vi "UI_AutoRefresh_Do.vi"(8 "error in (no error)":errorcluster, 9 "Parameters":T1={"Write TipStrips with details (T)"=TRUE, "Write Captions with UserLabels (T)"=TRUE, "Mode (ind only)"=enum."Indicators only", "Enable nested stream (T)"=TRUE}, 10 "Databox_sealed":refnum<class "Databox_sealed.lvclass">, 11 "LiveDatActor in":refnum<class "LiveDatActor.lvclass">) -> (0 "error out":errorcluster, 3 "LiveDatActor out":refnum<class "LiveDatActor.lvclass">)   [LabVIEW 2020, in "LiveDatActor.lvlib" / "LiveDatActor.lvclass"]
doc: "Enable nested stream : Permet le routage de la databox vers les nested UIA de l'acteur. On peut couper ce ruissellement si les nested n'ont pas besoin de databox pour optimiser le programme."
uses:
  LiveDatActor.lvclass
  support/UI_Actor.lvlibp/UI_Actor/ctl_AR_Parameters.ctl
  support/UI_Actor.lvlibp/UI_Actor/ctl_AR_Mode.ctl
  support/Databox.lvlibp/Databox_sealed/Databox_sealed.lvclass
  LiveDatActor.lvclass/LiveDatActor.ctl
  support/Databox.lvlibp/TypesTools/Data/Read Time.vi
  support/UI_Actor.lvlibp/UI_Actor/UI_Actor.lvclass
  support/Databox.lvlibp/TypesTools/Data/Data.lvclass
  D:/Projets/STEP AT/Bahamut/support/UI_Actor.lvlibp/UI_Actor/UI_Actor.lvclass
  D:/Projets/STEP AT/Bahamut/support/Actor Framework.lvlibp/1abvi3w/vi.lib/ActorFramework/Actor/Actor.lvclass
  D:/Projets/STEP AT/Bahamut/D&Cs/LiveDatActor/LiveDatActor/LiveDatActor.lvclass
  support/Databox.lvlibp/Databox/Databox.lvclass
  D:/Projets/STEP AT/Bahamut/support/Databox.lvlibp/Databox/Databox.lvclass
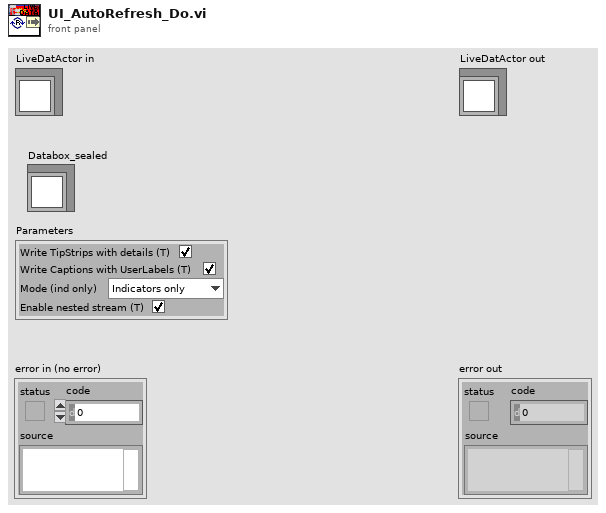
[diagram p1: front panel]
types:
  T1 = typedef "UI_Actor.lvlibp/UI_Actor.lvclass/ctl_AR_Parameters.ctl" = cluster{"Write TipStrips with details (T)":bool, "Write Captions with UserLabels (T)":bool, "Mode (ind only)":T2, "Enable nested stream (T)":bool}
  T2 = typedef "UI_Actor.lvlibp/UI_Actor.lvclass/ctl_AR_Mode.ctl" = enum16{"Controls only", "Indicators only", "All"}
  T3 = cluster{"Name":string, "Data":refnum<class "Data.lvclass">[]}[]
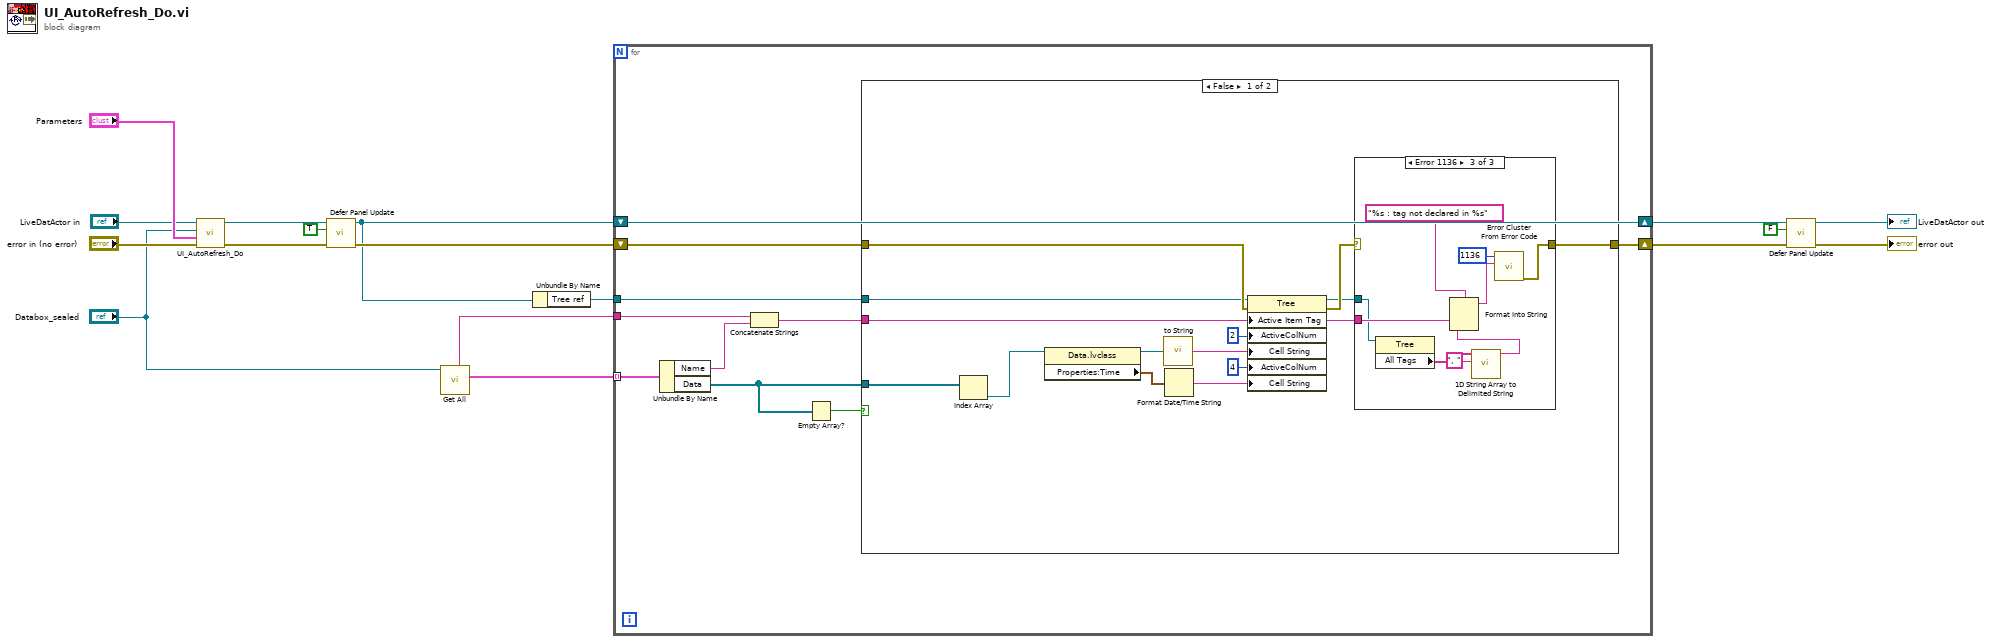
[diagram p0: block diagram]
diagram:
  n1 = call-parent "UI_AutoRefresh_Do.vi"("error in (no error)"="error in (no error)", "Parameters"="Parameters", "Databox_sealed"="Databox_sealed", "UI_Actor in"="LiveDatActor in") -> ("error out"=w11:errorcluster, "UI_Actor out"=w12:refnum<class "LiveDatActor.lvclass">)  [unwired: 6 in]
  n2 = call "Defer Panel Update.vi"("error in (no error)"=w11, "Defer Panel Updates"=TRUE, "UI_Actor in"=w12) -> ("error out"=w10:errorcluster, "UI_Actor out"=w9:refnum<class "LiveDatActor.lvclass">)  [unwired: 7 in]
  n3 = call "Get All.vi"("Databox in"="Databox_sealed") -> ("Names and data"=w2:T3, "Builder name"=w1:string)  [unwired: 5 in, 4 out]
  n4 = Unbundle By Name(w9) -> ("Tree ref"=w4:refnum<vi>)
  n5 = for {
    tunnel: w4 -> [w25]
    shift-right: [w27] -> w6
    shift-left: w9 -> [w27]
    shift-right: [w24] -> w8
    shift-left: w10 -> [w26]
    tunnel: w2 -> [w23] mode=indexing
    tunnel: w1 -> [w21]
    n6 = Unbundle By Name(w23) -> ("Name"=w20:string, "Data"=w19:refnum<class "Data.lvclass">[])
    n7 = Concatenate Strings(w21, w20) -> (w22:string)
    n8 = Empty Array?(array=w19) -> (empty?=w18:bool)
    n9 = case shown="False" w18 {
      tunnel: w26 -> [w41 w53]
      tunnel: w25 -> [w40 _]
      tunnel: [w39 w53] -> w24
      tunnel: w22 -> [w31 _]
      tunnel: w19 -> [w28 _]
      frame False {
        n10 = Index Array(array=w28) -> (element=w29:refnum<class "Data.lvclass">)  [unwired: 1 in]
        n11 = property class="Data.lvclass"(reference=w29) -> (reference out=w38:refnum<class "Data.lvclass">, "Properties:Time"=w34:timestamp)  [unwired: 1 in, 1 out]
        n12 = call "to String.vi"("Data"=w38) -> ("String"=w35:string)
        n13 = Format Date/Time String(seconds (now)=w34) -> (date/time string=w33:string)  [unwired: 2 in]
        n14 = property class="Tree"(reference=w40, error in=w41, "Active Item Tag"=w31, "ActiveColNum"=2 ("Active Cell:Active Column Number"), "Cell String"=w35, "ActiveColNum"=4 ("Active Cell:Active Column Number"), "Cell String"=w33) -> (reference out=w30:refnum<vi>, error out=w32:errorcluster)
        n15 = case shown="Error 1136" w32 {
          selector: w32 -> [w42 w43 _]
          tunnel: [w42 w43 w52] -> w39
          tunnel: w31 -> [_ _ w50]
          tunnel: w30 -> [_ _ w47]
          frame No Error {
          }
          frame Default {
          }
          frame Error {
            n16 = property class="Tree"(reference=w47) -> ("All Tags"=w46:string[])  [unwired: 1 in, 2 out]
            n17 = call <vilib>:"1D String Array to Delimited String.vi"("delimiter"=", ", "string array"=w46) -> ("delimited string"=w45:string)  [unwired: 9 in]
            n18 = Format Into String(format string="%s : tag not declared in %s", w50, w45) -> (resulting string=w48:string)  [unwired: 2 in, 1 out]
            n19 = call <vilib>:"Error Cluster From Error Code.vi"("error message (\"\")"=w48, "error code (0)"=1136) -> ("error out"=w52:errorcluster)  [unwired: 7 in]
          }
        }
      }
      frame True {
      }
    }
  }
  n20 = call "Defer Panel Update.vi"("error in (no error)"=w8, "Defer Panel Updates"=FALSE, "UI_Actor in"=w6) -> ("error out"=→"error out":errorcluster, "UI_Actor out"=→"LiveDatActor out":refnum<class "LiveDatActor.lvclass">)  [unwired: 7 in]
